vi "GetRemoteIP.vi"(8 "error in (no error)":errorcluster, 11 "SM1000-control in":T1) -> (0 "error out":errorcluster, 2 "Remote IP":string, 3 "SM1000-control out":T1)   [LabVIEW 2013, in "EC1000-control.lvlib" / "SM1000-control.lvclass"]
doc: "Returns the IP address of the LAN stream host that has control of the EC1000.\n\nIf no host has control, the address \"0.0.0.0\" is returned.\n\nCommand: \"GetRemoteIP\" or 9\nReturns: <[0-9].[0-9].[0-9].[0-9]>"
uses:
  SM1000-control.lvclass
  Object-reference.ctl
  SM1000-control.lvclass/SM1000-control.ctl
  Custom-errors.ctl
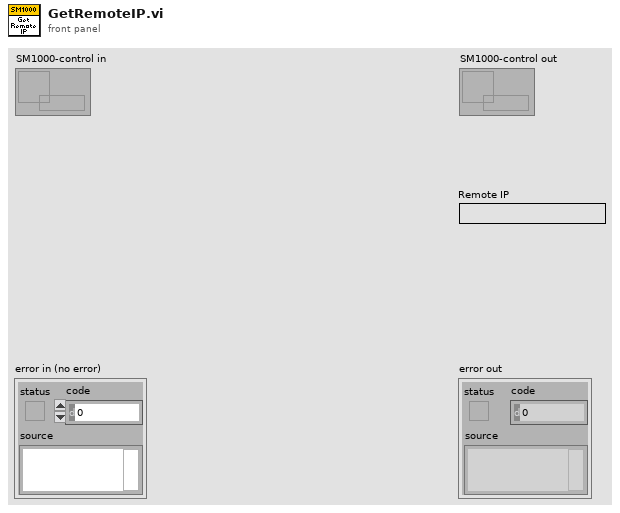
[diagram p1: front panel]
types:
  T1 = typedef "EC1000-control.lvlib/SM1000-control.lvclass/Object-reference.ctl" = refnum<data-value>
  T2 = typedef "EC1000-control.lvlib/SM1000-control.lvclass/Custom-errors.ctl" = enum16{"No error", "Not implemented", "Command not recognized", "Invalid input", "No connection", "Timeout", "Resource not loaded"}
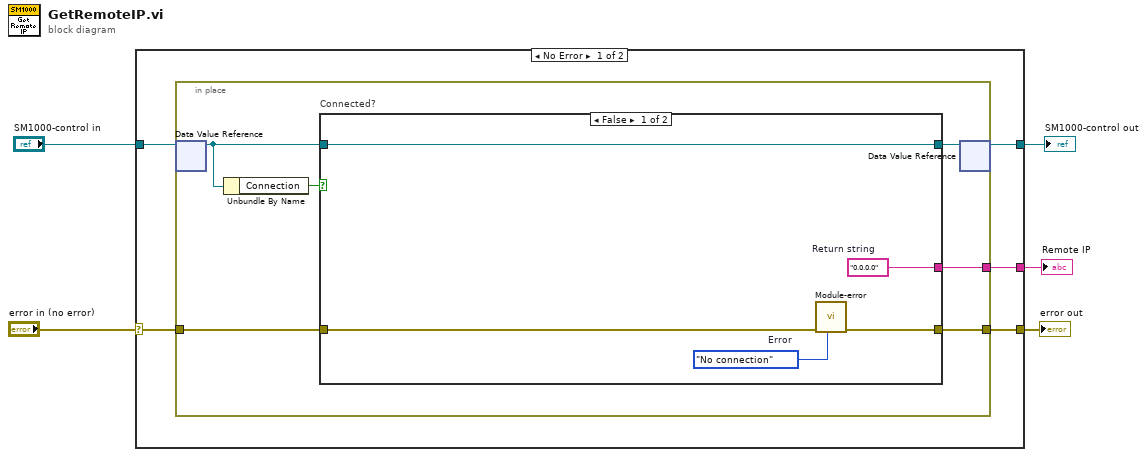
[diagram p0: block diagram]
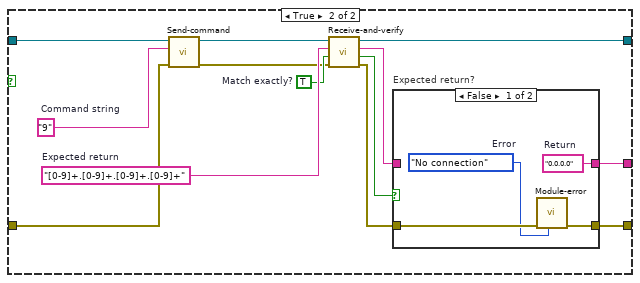
[diagram p2: hidden frame]
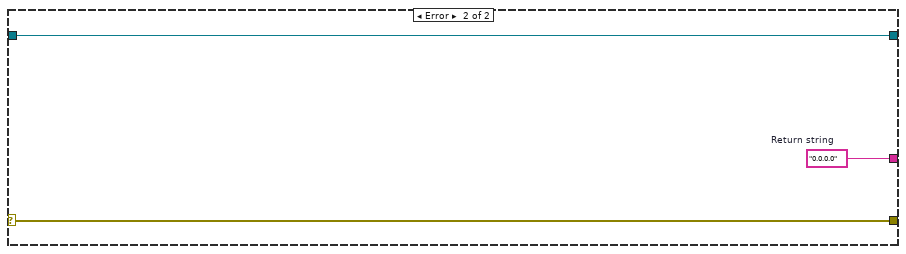
[diagram p4: hidden frame]
diagram:
  n1 = case shown="No Error" "error in (no error)" {
    selector: "error in (no error)" -> [w8 w43]
    tunnel: [w7 w43] -> w4
    tunnel: [w9 w42] -> w2
    tunnel: "SM1000-control in" -> [w10 w42]
    tunnel: [w6 w41] -> w1
    frame No Error {
      n2 = in-place {
        in-place-border: w8 -> [w16]
        in-place-border: [w13] -> w7
        in-place-border: [w11] -> w6
        n3 = in-place-dvr #1(w10) -> (w14:refnum<class "SM1000-control.lvclass">)  [unwired: 1 out]
        n4 = Unbundle By Name(w14) -> ("Connection"=w15:bool)
        n5 = case "Connected?" shown="False" w15 {
          tunnel: w16 -> [w21 w26]
          tunnel: w14 -> [w19 w34]
          tunnel: [w20 w24] -> w13
          tunnel: [w19 w23] -> w12
          tunnel: [w18 w22] -> w11
          frame False {
            w17 = Custom-errors."No connection"  # Error
            w18 = "0.0.0.0"  # Return string
            n6 = call "Module-error.vi"("Error"=w17, "error in (no error)"=w21) -> ("error out"=w20:errorcluster)  [unwired: 9 in]
          }
          frame True {
            w30 = TRUE  # Match exactly?
            w31 = "[0-9]+.[0-9]+.[0-9]+.[0-9]+"  # Expected return
            w32 = "9"  # Command string
            n7 = call "Send-command.vi"("error in (no error)"=w26, "Command string"=w32, "SM1000-control in"=w34) -> ("error out"=w29:errorcluster, "SM1000-control out"=w33:refnum<class "SM1000-control.lvclass">)  [unwired: 7 in]
            n8 = call "Receive-and-verify.vi"("error in (no error)"=w29, "Match exactly?"=w30, "Expected return string"=w31, "SM1000-control in"=w33) -> ("error out"=w25:errorcluster, "Verified?"=w28:bool, "Return string"=w27:string, "SM1000-control out"=w23:refnum<class "SM1000-control.lvclass">)  [unwired: 4 in]
            n9 = case "Expected return?" shown="False" w28 {
              tunnel: w27 -> [_ w40]
              tunnel: w25 -> [w37 w39]
              tunnel: [w36 w39] -> w24
              tunnel: [w38 w40] -> w22
              frame False {
                w35 = Custom-errors."No connection"  # Error
                w38 = "0.0.0.0"  # Return
                n10 = call "Module-error.vi"("Error"=w35, "error in (no error)"=w37) -> ("error out"=w36:errorcluster)  [unwired: 9 in]
              }
              frame True {
              }
            }
          }
        }
        n11 = in-place-dvr #1(w12) -> (w9:T1)  [unwired: 1 out]
      }
    }
    frame Error {
      w41 = "0.0.0.0"  # Return string
    }
  }
  "error out" <- w4
  "SM1000-control out" <- w2
  "Remote IP" <- w1
